vi "RSZVB Delete Group Of Measured Ports.vi"(8 "error in (no error)":errorcluster {"code" format="%.0x"}, 9 "Group (1)":i32=1, 10 "Channel (1)":i32=1, 11 "VISA session":refnum<visa-resource-name>) -> (0 "error out":errorcluster {"code" format="%.0x"}, 3 "dup VISA session":refnum<visa-resource-name>)   [LabVIEW 2011]
doc: "This VI dissolves a group of measured ports.\n\nRemote-control command(s):\nSOURce<Ch>:GROup<group_no>:CLEar"
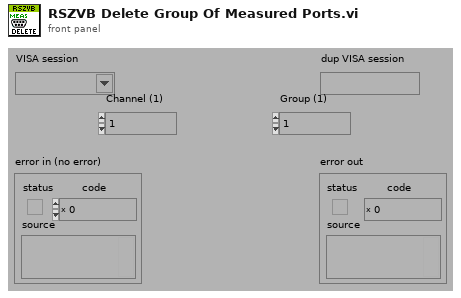
[diagram p1: front panel]
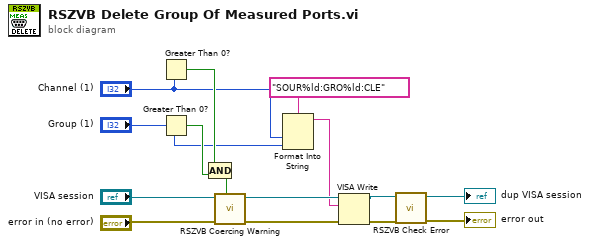
[diagram p0: block diagram]
diagram:
  n1 = Greater Than 0?(x="Channel (1)") -> (x > 0?=w9:bool)
  n2 = Greater Than 0?(x="Group (1)") -> (x > 0?=w10:bool)
  n3 = Compound Arithmetic op=AND(w9, w10) -> (w12:bool)
  n4 = call "RSZVB Coercing Warning.vi"("In Range?"=w12, "error in (no error)"="error in (no error)", "VISA session"="VISA session") -> ("error out"=w13:errorcluster, "dup VISA session"=w14:refnum<visa-resource-name>)  [unwired: 7 in]
  n5 = Format Into String(format string="SOUR%ld:GRO%ld:CLE", "Channel (1)", "Group (1)") -> (resulting string=w11:string)  [unwired: 2 in, 1 out]
  n6 = VISA Write(VISA resource name=w14, write buffer=w11, error in (no error)=w13) -> (VISA resource name out=w7:refnum<visa-resource-name>, error out=w6:errorcluster)  [unwired: 1 out]
  n7 = call "RSZVB Check Error.vi"("error in (no error)"=w6, "VISA session"=w7) -> ("error out"=→"error out":errorcluster, "dup VISA session"=→"dup VISA session":refnum<visa-resource-name>)  [unwired: 8 in]
